vi "Zellen einfaerben.vi"(7 "Löschen":bool, 10 "Färben":bool[](array[boolean]), 11 "Tabellenref.":refnum<vi>) -> ()   [LabVIEW 2020, in "Linearisierung v2.lvlib" / "Linearity verification 1065-307.lvlib"]
uses:
  Linearity verification 1065-307.lvlib
  <vilib>/Utility/miscctls.llb/LVRowAndColumnTypeDef.ctl
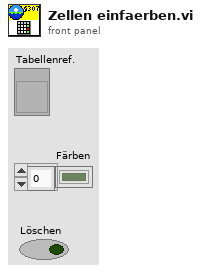
[diagram p1: front panel]
types:
  T1 = typedef "LVRowAndColumnTypeDef.ctl" = cluster{"Row":i32, "Column":i32}
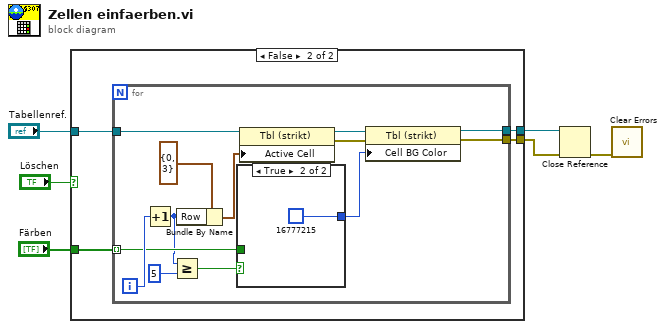
[diagram p0: block diagram]
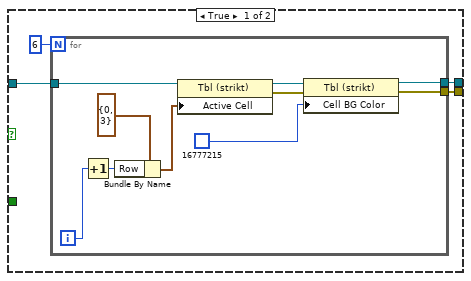
[diagram p2: hidden frame]
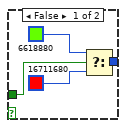
[diagram p3: hidden frame]
diagram:
  n1 = case shown="False" "Löschen" {
    tunnel: "Tabellenref." -> [w10 w24]
    tunnel: "Färben" -> [_ w23]
    tunnel: [w9 w22] -> w4
    tunnel: [w8 w21] -> w3
    frame True {
      n2 = for {
        N: 6 -> [_]
        tunnel: w10 -> [w20]
        tunnel: [w13] -> w9
        tunnel: [w12] -> w8
        i -> [w14]
        n3 = Increment(x=w14) -> (x+1=w15:i32)
        n4 = Bundle By Name(cluster=T1 {"Row"=0, "Column"=3} ("Aktive Zelle:Aktive Zelle"), "Row"=w15) -> (w18:T1)
        n5 = property class="Tbl (strikt)"(reference=w20, "Active Cell"=w18) -> (reference out=w17:refnum<vi>, error out=w16:errorcluster)  [unwired: 1 in]
        n6 = property class="Tbl (strikt)"(reference=w17, error in=w16, "Cell BG Color"=u32 16777215) -> (reference out=w13:refnum<vi>, error out=w12:errorcluster)
      }
    }
    frame False {
      n7 = for {
        tunnel: w24 -> [w37]
        tunnel: w23 -> [w30] mode=indexing
        tunnel: [w29] -> w22
        tunnel: [w28] -> w21
        i -> [w31]
        n8 = Increment(x=w31) -> (x+1=w27:i32)
        n9 = Greater Or Equal?(x=w27, y=5) -> (x >= y?=w25:bool)
        n10 = Bundle By Name(cluster=T1 {"Row"=0, "Column"=3} ("Aktive Zelle:Aktive Zelle"), "Row"=w27) -> (w35:T1)
        n11 = case shown="True" w25 {
          tunnel: [w39 u32 16777215] -> w32
          tunnel: w30 -> [w38 _]
          frame False {
            n12 = Select(t=u32 6618880, s=w38, f=u32 16711680) -> (s? t:f=w39:u32)
          }
          frame True {
          }
        }
        n13 = property class="Tbl (strikt)"(reference=w37, "Active Cell"=w35) -> (reference out=w34:refnum<vi>, error out=w33:errorcluster)  [unwired: 1 in]
        n14 = property class="Tbl (strikt)"(reference=w34, error in=w33, "Cell BG Color"=w32) -> (reference out=w29:refnum<vi>, error out=w28:errorcluster)
      }
    }
  }
  n15 = Close Reference(reference=w4, error in (no error)=w3) -> (error out=w2:errorcluster)
  n16 = call <vilib>:"Clear Errors.vi"("error in (no error)"=w2) -> ()  [unwired: 5 in, 2 out]
